vi "field and type to key.vi"(10 "wire type":T1, 11 "field number":u64) -> (3 "key":u64)   [LabVIEW 2013, in "protocol buffers encoder.lvlib"]
uses:
  protocol buffers encoder.lvlib
  wire type.ctl
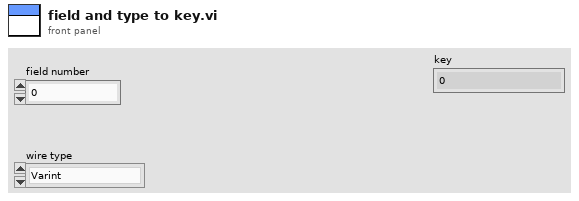
[diagram p1: front panel]
types:
  T1 = typedef "protocol buffers encoder.lvlib/wire type.ctl" = enum8{"Varint", "64 bit", "Length Delimited", "Start Group", "End Group", "32 bit"}
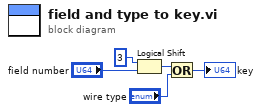
[diagram p0: block diagram]
diagram:
  n1 = Logical Shift(y=i16 3, x="field number") -> (x << y=w3:u64)
  n2 = Or(x=w3, y="wire type") -> (x .or. y?=→"key":u64)
